vi "GEA2 Send and Receive Message.vi"(0 "GEA2 Reference In":refnum<k24>, 1 "Input Data":T1={"Source"=228, "Destination"=37, "Command"=158, "Message"=""} {"Command" format="%02x"; "Destination" format="%02x"; "Source" format="%02x"}, 2 "Read Timeout (ms)":u32=500, 3 "# of Retries":i32=3, 5 "Expected Command":string=".*", 7 "Expected Data":string=".*", 9 "GEA2 Event Registration":refnum<event-registration>, 11 "Error In":errorcluster) -> (4 "GEA2 Reference Out":refnum<k24>, 6 "Raw Data Out":string, 8 "Converted Data Out":T2 {"CRC" format="%04x"; "Length" format="%02x"; "Command" format="%02x"; "Destination" format="%02x"; "Source" format="%02x"}, 10 "Event Registration Out":refnum<event-registration>, 14 "Raw Data":string, 15 "Error Out":errorcluster)   [LabVIEW 2016, in "GEA2_Toolkit.lvlib"]
doc: "This VI sends and receives data across the GEA2 bus. The VI waits for the expected responses (filtered by the expected command / data fields) or until the timeout occurs."
uses:
  library/GEA2_Toolkit.lvlib
  type defs/Data Out.ctl
  type defs/Data In.ctl
  C:/Technology Lab/NI-2010/Trunk/Utility/LabVIEW GEA2 Toolkit v1.0.0.0/Appliance.NET/GeaCommunication.dll
  Appliance.NET/GeaCommunication.dll
panel:
  out "All Data":string
  out "Interations":i32=2 format="%x"
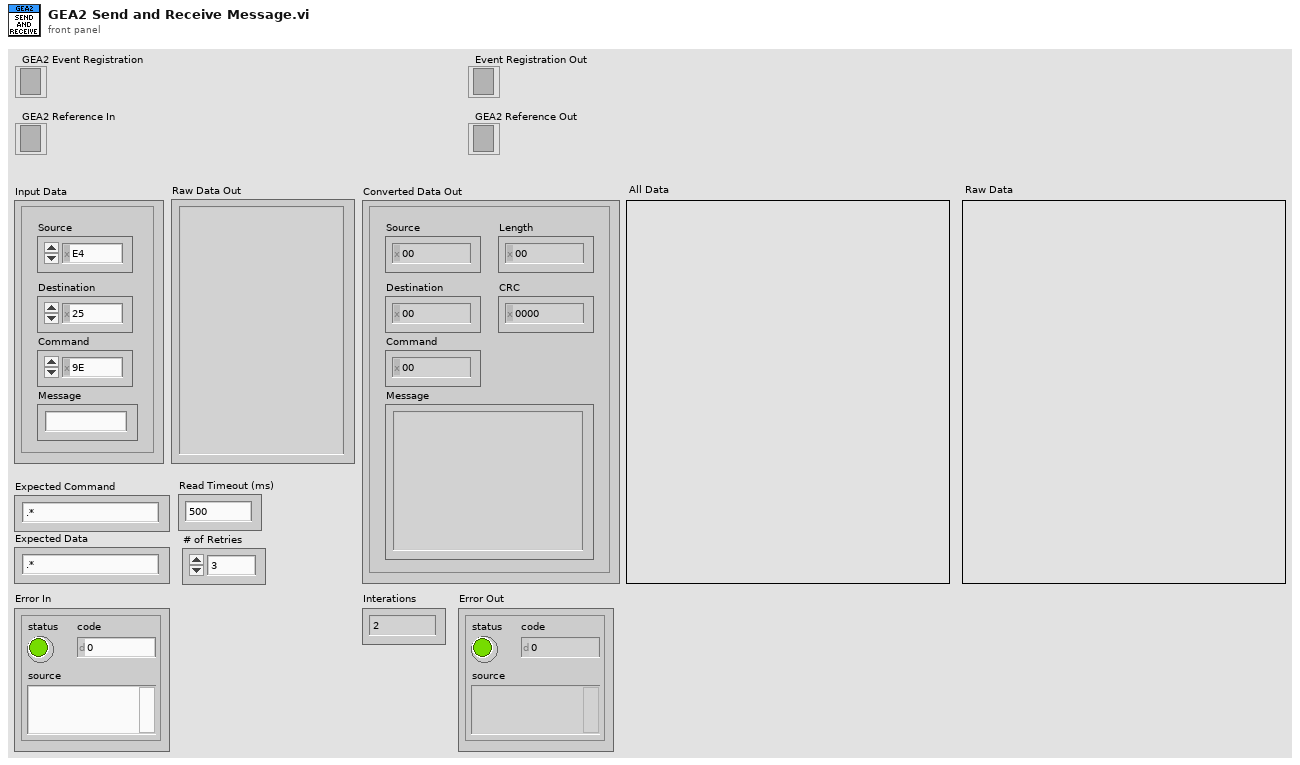
[diagram p1: front panel]
types:
  T1 = typedef "GEA2_Toolkit.lvlib/Data In.ctl" = cluster{"Source":u8, "Destination":u8, "Command":u8, "Message":string}
  T2 = typedef "GEA2_Toolkit.lvlib/Data Out.ctl" = cluster{"Source":u8, "Destination":u8, "Command":u8, "Length":u8, "CRC":u16, "Message":string}
  T3 = typedef "eventsource.ctl" = u32
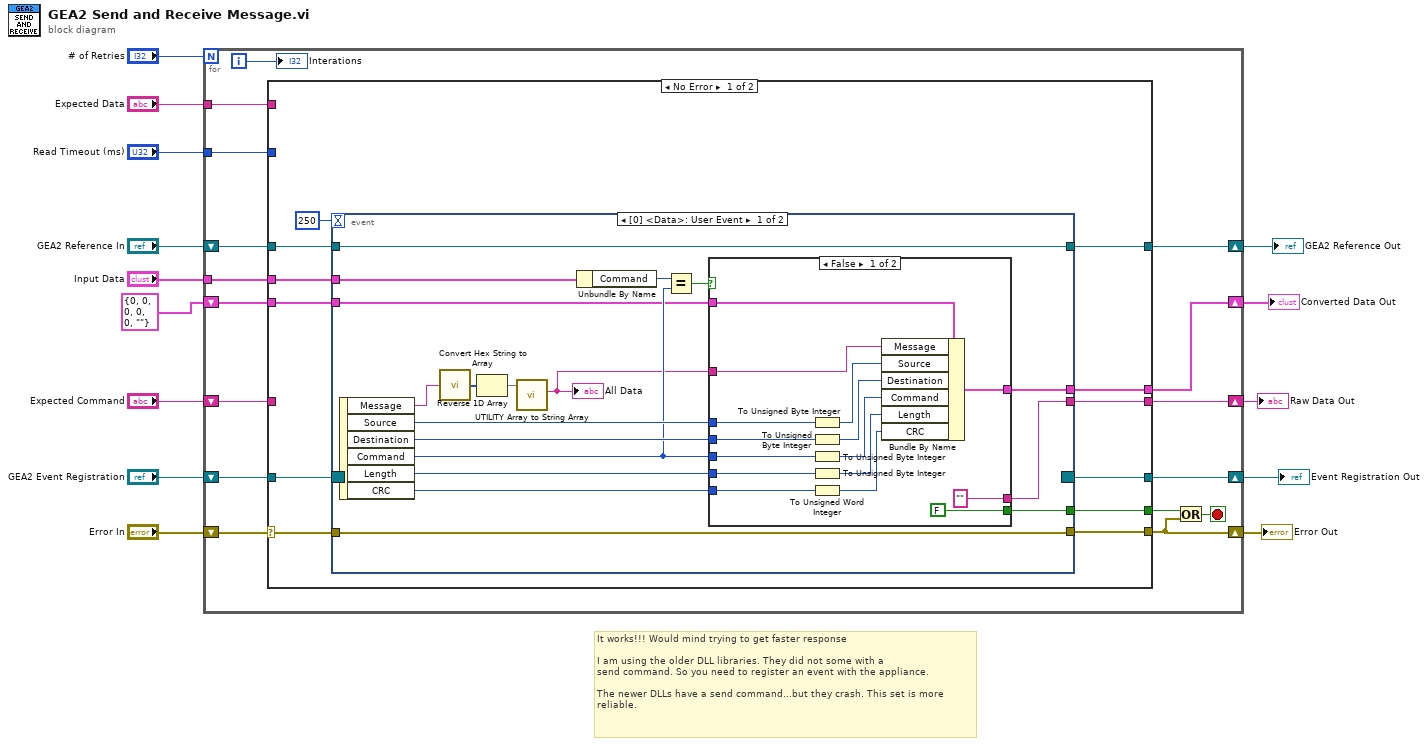
[diagram p0: block diagram]
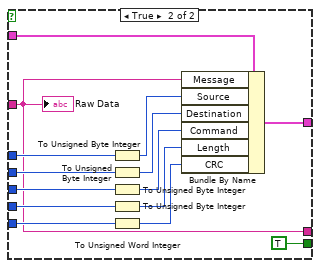
[diagram p2: hidden frame]
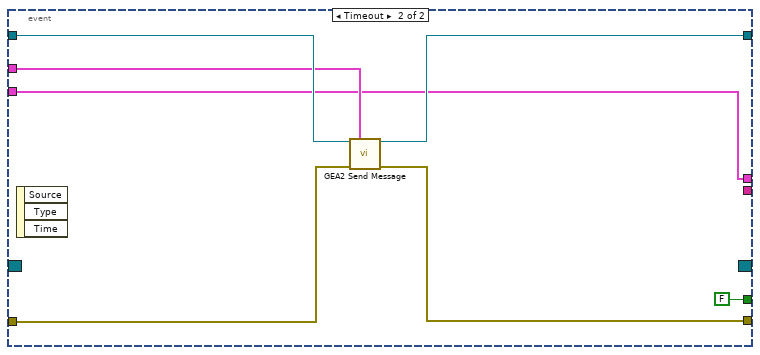
[diagram p3: hidden frame]
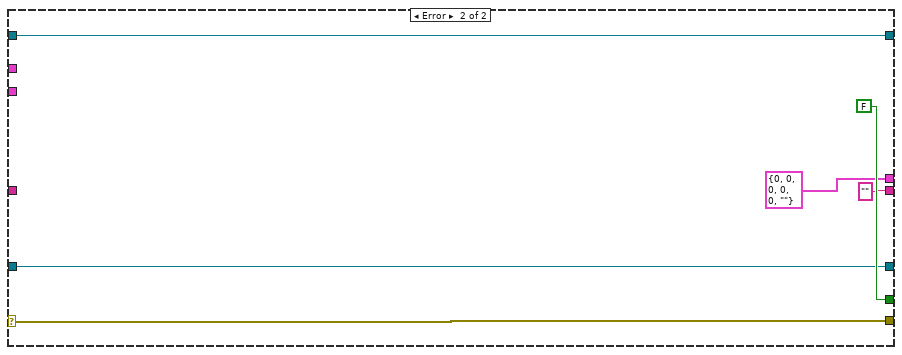
[diagram p4: hidden frame]
diagram:
  # "It works!!! Would mind trying to get faster response\n\nI am using the older DLL libraries. They did not some with a \nsend command. So you need to register an event with the appliance.\n\nThe newer DLLs have a send command...but they crash. This set is more\nreliable."
  n1 = for {
    N: "# of Retries" -> [_]
    tunnel: "Read Timeout (ms)" -> [w29]
    tunnel: "Expected Data" -> [w26]
    tunnel: "Input Data" -> [w24]
    shift-right: [w20] -> w3
    shift-left: "Error In" -> [w30]
    shift-right: [w28] -> w12
    shift-left: "Expected Command" -> [w25]
    shift-right: [w22] -> w6
    shift-left: "GEA2 Reference In" -> [w23]
    shift-right: [w16] -> w2
    shift-left: "GEA2 Event Registration" -> [w21]
    shift-right: [w27] -> w11
    shift-left: T2 {"Source"=0, "Destination"=0, "Command"=0, "Length"=0, "CRC"=0, "Message"=""} ("Coverted Data Out") -> [w15]
    i -> [w17]
    stop <- w18 stop-if-true
    n2 = case shown="No Error" w30 {
      selector: w30 -> [w37 w101]
      tunnel: w23 -> [w40 w102]
      tunnel: [w35 T2 {"Source"=0, "Destination"=0, "Command"=0, "Length"=0, "CRC"=0, "Message"=""} ("Coverted Data Out")] -> w27
      tunnel: [w39 w102] -> w22
      tunnel: [w38 w101] -> w20
      tunnel: w29 -> [_ _]
      tunnel: [w34 "" ("Message")] -> w28
      tunnel: w26 -> [_ _]
      tunnel: w25 -> [_ _]
      tunnel: w24 -> [w41 _]
      tunnel: w21 -> [w36 w97]
      tunnel: [w33 FALSE] -> w19
      tunnel: [w32 w97] -> w16
      tunnel: w15 -> [w31 _]
      frame No Error {
        n3 = event shown="[0] <Data>: User Event" {
          selector: w36 -> [_ _]
          dyn-events: [_ _] -> w32
          timeout: 250 -> [_ _]
          tunnel: w37 -> [w60 w96]
          tunnel: [w60 w95] -> w38
          tunnel: w41 -> [w57 w92]
          tunnel: w40 -> [w56 w94]
          tunnel: [w56 w93] -> w39
          tunnel: [w55 w90] -> w35
          tunnel: [w48 _] -> w34
          tunnel: [w49 FALSE] -> w33
          tunnel: w31 -> [w47 w90]
          event User Event {
            n4 = event-data() -> ("Message"=w44:string, "Source"=w54:T3, "Destination"=w53:u8, "Command"=w52:u8, "Length"=w51:u8, "CRC"=w50:u16)  [unwired: 1 in]
            n5 = call "Convert Hex String to Array.vi"("Hex String In"=w44) -> ("Hex Array Out"=w46:u8[])  [unwired: 14 in]
            n6 = Reverse 1D Array(array=w46) -> (reversed array=w45:u8[])
            n7 = call "UTILITY Array to String Array.vi"("Hex Array Out"=w45) -> ("String"=w43:string)  [unwired: 9 in, 1 out]
            "All Data" <- w43
            n8 = Unbundle By Name(w57) -> ("Command"=w59:u8)
            n9 = Equal?(x=w59, y=w52) -> (x = y?=w58:bool)
            n10 = case shown="False" w58 {
              tunnel: w43 -> [w63 w77]
              tunnel: [w61 w84] -> w55
              tunnel: w54 -> [w64 w83]
              tunnel: w53 -> [w65 w82]
              tunnel: w52 -> [w66 w81]
              tunnel: w51 -> [w67 w80]
              tunnel: w50 -> [w68 w79]
              tunnel: [FALSE TRUE] -> w49
              tunnel: ["" ("Message") w77] -> w48
              tunnel: w47 -> [w62 w76]
              frame False {
                n11 = To Unsigned Byte Integer(number=w64) -> (unsigned 8bit integer=w70:u8)
                n12 = To Unsigned Byte Integer(number=w65) -> (unsigned 8bit integer=w69:u8)
                n13 = To Unsigned Byte Integer(number=w66) -> (unsigned 8bit integer=w71:u8)
                n14 = To Unsigned Byte Integer(number=w67) -> (unsigned 8bit integer=w72:u8)
                n15 = To Unsigned Word Integer(number=w68) -> (unsigned 16bit integer=w73:u16)
                n16 = Bundle By Name(cluster=w62, "Message"=w63, "Source"=w70, "Destination"=w69, "Command"=w71, "Length"=w72, "CRC"=w73) -> (w61:T2)
              }
              frame True {
                n17 = To Unsigned Byte Integer(number=w83) -> (unsigned 8bit integer=w86:u8)
                n18 = To Unsigned Byte Integer(number=w82) -> (unsigned 8bit integer=w85:u8)
                n19 = To Unsigned Byte Integer(number=w81) -> (unsigned 8bit integer=w87:u8)
                n20 = To Unsigned Byte Integer(number=w80) -> (unsigned 8bit integer=w88:u8)
                n21 = To Unsigned Word Integer(number=w79) -> (unsigned 16bit integer=w89:u16)
                n22 = Bundle By Name(cluster=w76, "Message"=w77, "Source"=w86, "Destination"=w85, "Command"=w87, "Length"=w88, "CRC"=w89) -> (w84:T2)
                "Raw Data" <- w77
              }
            }
          }
          event Timeout {
            n23 = event-data() -> ()  [unwired: 1 in, 3 out]
            n24 = call "GEA2 Send Message.vi"("GEA2 Reference In"=w94, "Input Data"=w92, "Error In"=w96) -> ("GEA2 Reference Out"=w93:refnum<k24>, "Error Out"=w95:errorcluster)  [unwired: 11 in]
          }
        }
      }
      frame Error {
      }
    }
    n25 = Or(x=w19, y=w20) -> (x .or. y?=w18:bool)
    "Interations" <- w17
  }
  "Raw Data Out" <- w12
  "Error Out" <- w3
  "Converted Data Out" <- w11
  "GEA2 Reference Out" <- w6
  "Event Registration Out" <- w2
